vi "Init.vi"(8 "error in (no error)":errorcluster, 10 "server cfg":T1={"API Root"="", "verify server"=FALSE, "Version (no version)"="", "Port (protocol specific)"=0, "Base URL"="", "Auth type"=enum."Token", "Auth string"="", "timeout (10000)"=10000, "Token preamble (Token)"="", "Token empty preamble (False)"=FALSE, "Token header key (Authorization)"=""}, 11 "ByteGSAPIBase in":refnum<class "ByteGSAPIBase.lvclass">) -> (0 "error out":errorcluster, 3 "ByteGSAPIBase out":refnum<class "ByteGSAPIBase.lvclass">)   [LabVIEW 2019, in "ByteGSWebAPI.lvlib" / "ByteGSAPIBase.lvclass"]
doc: "Initialize the api connection based on a server cfg cluster"
uses:
  ByteGSAPIBase.lvclass
  <vilib>/Bytelabs/ByteREST/CfgLoaders/LoaderBase/ServerParams.ctl
  <vilib>/Bytelabs/ByteREST/ByteRESTClass/ByteRESTBase/Auth/Authentication_type.ctl
  ByteGSAPIBase.lvclass/ByteGSAPIBase.ctl
  <vilib>/Bytelabs/ByteREST/CfgLoaders/LoaderConstant/RESTLoaderConstant.lvclass/RESTLoaderConstant.ctl
  <vilib>/Bytelabs/ByteREST/CfgLoaders/LoaderConstant/RESTLoaderConstant.lvclass
  C:/Program Files (x86)/National Instruments/LabVIEW 2019/vi.lib/Bytelabs/ByteREST/CfgLoaders/LoaderBase/RESTLoaderBase.lvclass
  <vilib>/Bytelabs/ByteREST/ByteRESTClass/ByteRESTBase/RESTBase.lvclass
  <vilib>/Bytelabs/ByteREST/CfgLoaders/LoaderBase/RESTLoaderBase.lvclass
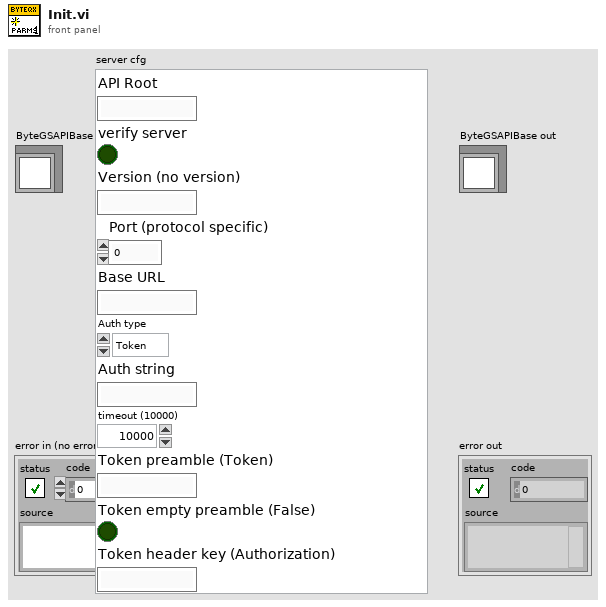
[diagram p1: front panel]
types:
  T1 = typedef "ByteREST.lvlib/RESTLoaderBase.lvclass/ServerParams.ctl" = cluster{"API Root":string, "verify server":bool, "Version (no version)":string, "Port (protocol specific)":u16, "Base URL":string, "Auth type":T2, "Auth string":string, "timeout (10000)":i32, "Token preamble (Token)":string, "Token empty preamble (False)":bool, "Token header key (Authorization)":string}
  T2 = typedef "ByteREST.lvlib/RESTBase.lvclass/Authentication_type.ctl" = enum16{"Token"}
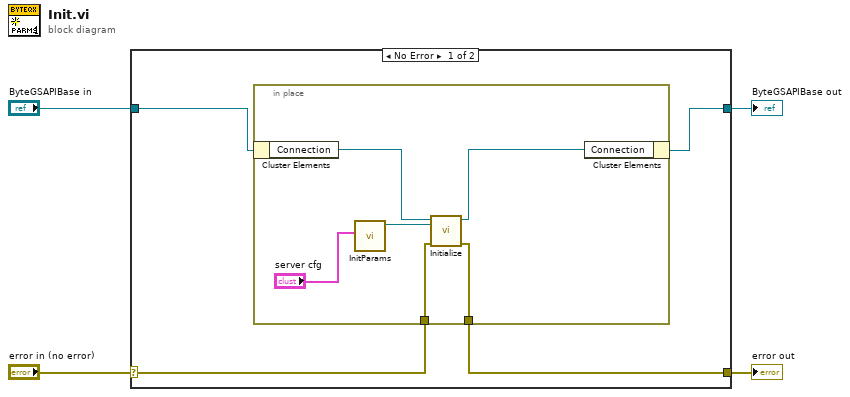
[diagram p0: block diagram]
diagram:
  n1 = case shown="No Error" "error in (no error)" {
    selector: "error in (no error)" -> [w6 w16]
    tunnel: [w5 w16] -> w3
    tunnel: [w7 w15] -> w1
    tunnel: "ByteGSAPIBase in" -> [w8 w15]
    frame No Error {
      n2 = in-place {
        in-place-border: w6 -> [w11]
        in-place-border: [w10] -> w5
        n3 = in-place-cluster #1(w8) -> ("Connection"=w14:refnum<class "RESTBase.lvclass">)
        n4 = call <vilib>:"InitParams.vi"("Cluster"="server cfg") -> ("RESTLoaderConstant out"=w12:refnum<class "RESTLoaderConstant.lvclass">)  [unwired: 10 in]
        n5 = call-dynamic "Initialize.vi"("error in (no error)"=w11, "RESTLoader"=w12, "REST in"=w14) -> ("error out"=w10:errorcluster, "REST out"=w9:refnum<class "RESTBase.lvclass">)  [unwired: 7 in]
        n6 = in-place-cluster #1("Connection"=w9) -> (w7:refnum<class "ByteGSAPIBase.lvclass">)
      }
    }
    frame Error {
    }
  }
  "error out" <- w3
  "ByteGSAPIBase out" <- w1
